vi "setTheme.Font.vi"(10 "Font":T1, 11 "Filled Text Fields Actor in":refnum<class "Filled Text Fields Actor.lvclass">) -> (3 "Filled Text Fields Actor out":refnum<class "Filled Text Fields Actor.lvclass">)   [LabVIEW 2017, in "Filled Text Fields.lvlib" / "Filled Text Fields Actor.lvclass"]
uses:
  Filled Text Fields Actor.lvclass
  Theme/Theme.Font/Font.ctl
  Filled Text Fields Actor.lvclass/Filled Text Fields Actor.ctl
  Theme/Theme/setFont.vi
  Theme/Theme/Theme.lvclass
  Theme/Theme.Font/Theme.Font.lvclass
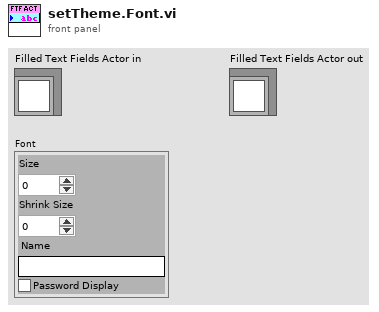
[diagram p1: front panel]
types:
  T1 = typedef "Theme.lvlib/Theme.Font.lvclass/Font.ctl" = cluster{"Size":u32, "Shrink Size":u32, "Name":string, "Password Display":bool}
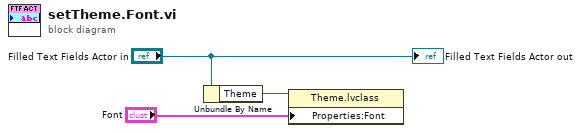
[diagram p0: block diagram]
diagram:
  n1 = Unbundle By Name("Filled Text Fields Actor in") -> ("Theme"=w2:refnum<class "Theme.lvclass">)
  n2 = property class="Theme.lvclass"(reference=w2, "Properties:Font"="Font") -> ()  [unwired: 1 in, 2 out]
  "Filled Text Fields Actor out" <- "Filled Text Fields Actor in"
